vi "Get Number of Sequences.vi"(8 "error in (no error)":errorcluster, 11 "VISA resource name":refnum<visa-resource-name>) -> (0 "error out":errorcluster, 2 "Number of sequences":i32, 3 "VISA resource name out":refnum<visa-resource-name>)   [LabVIEW 2020, in "QuPMXdriver.lvlib"]
doc: "Returns the actual number of sequences in multiplexer memory."
uses:
  QuPMXdriver.lvlib
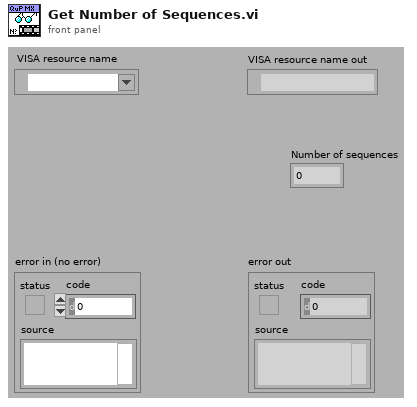
[diagram p1: front panel]
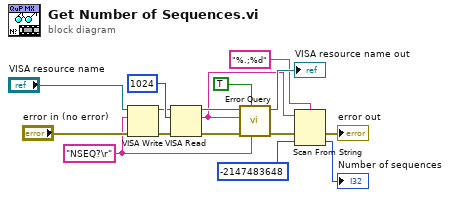
[diagram p0: block diagram]
diagram:
  w4 = "NSEQ?\r"
  n1 = VISA Write(VISA resource name="VISA resource name", write buffer=w4, error in (no error)="error in (no error)") -> (VISA resource name out=w11:refnum<visa-resource-name>, error out=w3:errorcluster)  [unwired: 1 out]
  n2 = VISA Read(VISA resource name=w11, byte count=u32 1024, error in (no error)=w3) -> (VISA resource name out=w10:refnum<visa-resource-name>, read buffer=w5:string, error out=w9:errorcluster)  [unwired: 1 out]
  n3 = call "Error Query.vi"("Last command"=w4, "Ignore empty sequence? (T)"=TRUE, "error in (no error)"=w9, "Read buffer"=w5, "VISA resource name"=w10) -> ("error out"=w7:errorcluster, "VISA resource name out"=→"VISA resource name out":refnum<visa-resource-name>)  [unwired: 5 in]
  n4 = Scan From String(format string="%.;%d", input string=w5, error in=w7, default 1=-2147483648 ("default value 1")) -> (error out=→"error out":errorcluster, output 1=→"Number of sequences":i32)  [unwired: 1 in, 2 out]
